vi "Prepare Response.vi"(8 "error in (no error)":errorcluster, 11 "PUBLISH in":refnum<class "PUBLISH.lvclass">) -> (0 "error out":errorcluster, 1 "response prepared?":bool, 2 "ControlPacket response":refnum<class "ControlPacket.lvclass">, 3 "PUBLISH out":refnum<class "PUBLISH.lvclass">)   [LabVIEW 2013, in "MQTT_Control_Packets.lvlib" / "PUBLISH.lvclass"]
uses:
  PUBLISH.lvclass
  ControlPacket/ControlPacket.lvclass
  ControlPacket/ControlPacket.lvclass/ControlPacket.ctl
  PUBACK/PUBACK.lvclass
  PUBREC/PUBREC.lvclass
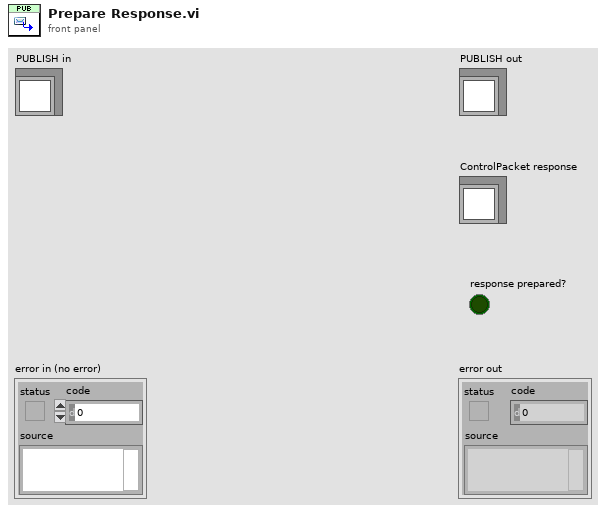
[diagram p1: front panel]
types:
  T1 = typedef "MQTT_Control_Packets.lvlib/ControlPacket.lvclass/QualityOfService -- enum.ctl" = enum16{"0 (At Most Once)", "1 (At Least Once)", "2 (Exactly Once)"}
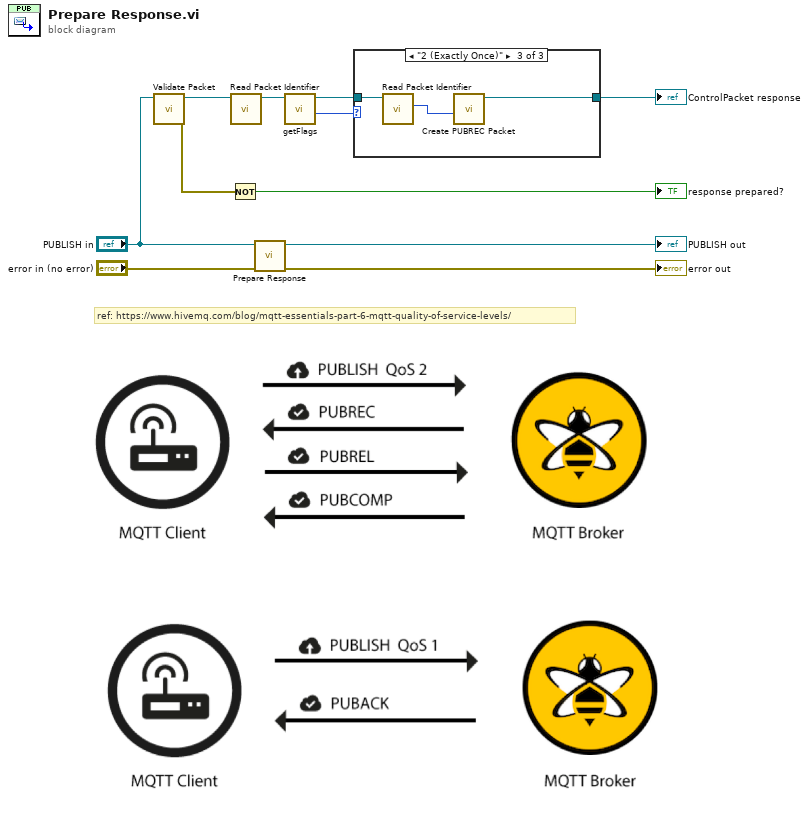
[diagram p0: block diagram]
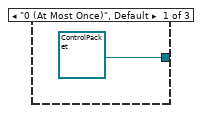
[diagram p2: hidden frame]
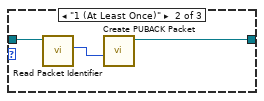
[diagram p3: hidden frame]
diagram:
  # "ref: https://www.hivemq.com/blog/mqtt-essentials-part-6-mqtt-quality-of-service-levels/"
  n1 = call "Validate Packet.vi"("ControlPacket in"="PUBLISH in") -> ("error out"=w7:errorcluster, "ControlPacket out"=w8:refnum<class "PUBLISH.lvclass">)  [unwired: 9 in]
  n2 = Not(x=w7) -> (.not. x?=→"response prepared?":bool)
  n3 = call "Read Packet Identifier.vi"("ControlPacket in"=w8) -> ("ControlPacket out"=w4:refnum<class "PUBLISH.lvclass">)  [unwired: 9 in, 1 out]
  n4 = call-parent "Prepare Response.vi"("error in (no error)"="error in (no error)", "ControlPacket in"="PUBLISH in") -> ("error out"=→"error out":errorcluster, "ControlPacket out"=→"PUBLISH out":refnum<class "PUBLISH.lvclass">)  [unwired: 6 in, 2 out]
  n5 = call-dynamic "getFlags.vi"("PUBLISH in"=w4) -> ("QoS"=w3:T1, "PUBLISH out"=w2:refnum<class "PUBLISH.lvclass">)  [unwired: 7 in, 2 out]
  n6 = case shown="\"2 (Exactly Once)\"" w3 {
    tunnel: w2 -> [_ w14 w17]
    tunnel: [refnum<class "ControlPacket.lvclass"> refnum ("MQTT_Control_Packets.lvlib:ControlPacket.lvclass") w15 w18] -> w1
    frame "0 (At Most Once)", Default {
    }
    frame "1 (At Least Once)" {
      n7 = call "Read Packet Identifier.vi"("ControlPacket in"=w14) -> ("Packet Identifier"=w13:u16)  [unwired: 9 in, 1 out]
      n8 = call "Create PUBACK Packet.vi"("Packet ID"=w13) -> ("PUBACK out"=w15:refnum<class "PUBACK.lvclass">)  [unwired: 9 in, 1 out]
    }
    frame "2 (Exactly Once)" {
      n9 = call "Read Packet Identifier.vi"("ControlPacket in"=w17) -> ("Packet Identifier"=w16:u16)  [unwired: 9 in, 1 out]
      n10 = call "Create PUBREC Packet.vi"("Packet ID"=w16) -> ("PUBREC out"=w18:refnum<class "PUBREC.lvclass">)  [unwired: 9 in, 1 out]
    }
  }
  "ControlPacket response" <- w1
